vi "ProducerConsumerData 1.vi"() -> ()   [LabVIEW 2017, in "Status Monitor Library.lvlib"]
doc: "Use this template to build a producer/consumer design pattern. Use this template when you need to execute a process, such as data analysis, when a data source, such as a triggered acquisition, produces data at an uneven rate and you need to execute the process when the data becomes available."
uses:
  Status Monitor Library.lvlib
  Communications/Communications Library.lvlib
panel:
  in  "Process Stop Button":bool
  out "Demuxing":bool
  out "Total Samples":i32
  out "Post-Buffered Samples":i32
  out "Pre-Buffered Samples":i32
  out "Device State":T1(ring)
  in  "timeout (ms)":i32
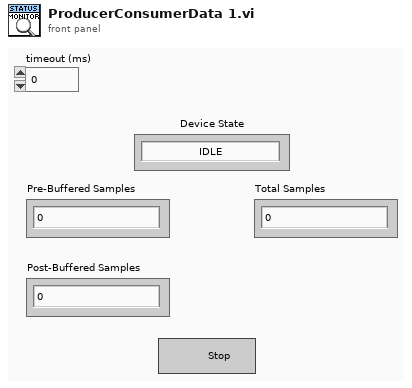
[diagram p1: front panel]
types:
  T1 = enum16{"IDLE", "ARM", "RUN_PRE-TRIGGER", "RUN_POST-TRIGGER", "POST_PROCESS", "CLEANUP"}
  T2 = typedef "Communications Library.lvlib/DTACQ Connection Data--Cluster.ctl" = cluster{"Description":string, "Address":string, "Port":u16, "timeout (ms)":i32, "Termination Character":string, "TCP Connection Reference":refnum<k5>, "Open Connection":bool}
  T3 = typedef "Communications Library.lvlib/DTACQ Module Carrier Status.ctl" = cluster{"DTACQ State":T4, "Pre-Trigger Samples":i32, "Post-Trigger Samples":i32, "Total Samples":i32, "Post Processing":bool}
  T4 = typedef "Communications Library.lvlib/DTACQ Status--Enum.ctl" = enum16{"IDLE", "ARM", "RUN_PRE-TRIGGER", "RUN_POST-TRIGGER", "POST_PROCESS", "CLEANUP"}
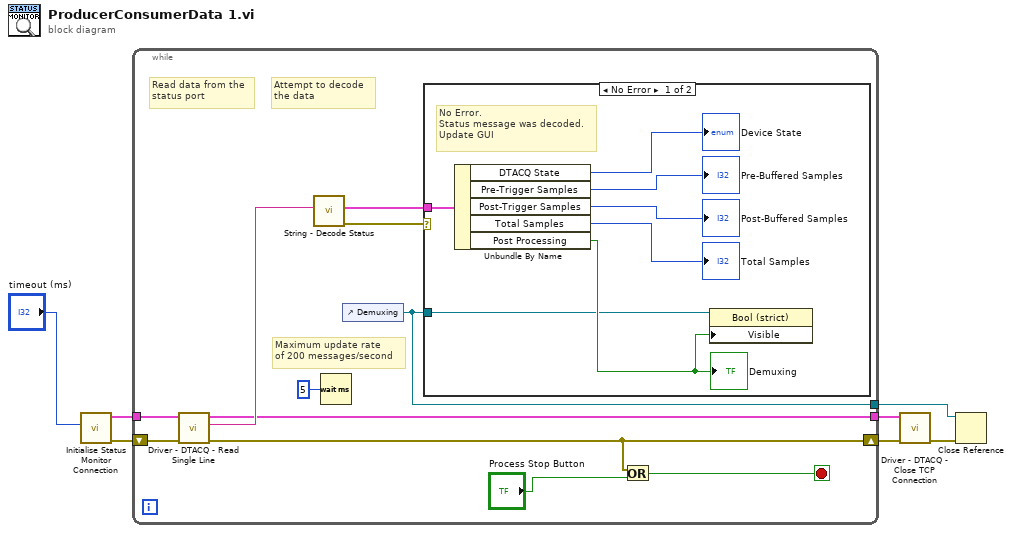
[diagram p0: block diagram]
diagram:
  n1 = call "Initialise Status Monitor Connection.vi"("timeout (ms)"="timeout (ms)") -> ("error out"=w5:errorcluster, "Status Connection Out"=w6:T2)  [unwired: 9 in]
  n2 = while {
    tunnel: w6 -> [w18]
    shift-right: [w13] -> w3
    shift-left: w5 -> [w16]
    tunnel: [w10] -> w4
    tunnel: [w9] -> w2
    stop <- w12 stop-if-true
    # "Maximum update rate\nof 200 messages/second"
    # "Attempt to decode\nthe data"
    # "Read data from the\nstatus port"
    n3 = call "Driver - DTACQ - Read Single Line.vi"("error in"=w16, "DTACQ Connection Data In"=w18) -> ("error out"=w13:errorcluster, "Read String"=w17:string, "DTACQ Connection Data Out"=w9:T2)  [unwired: 6 in, 1 out]
    n4 = call "String - Decode Status.vi"("Status Response String"=w17) -> ("error out"=w15:errorcluster, "Module Carrier Status"=w14:T3)  [unwired: 9 in]
    n5 = Wait (ms)(milliseconds to wait=u32 5) -> ()  [unwired: 1 out]
    n6 = control-ref of="Demuxing"() -> (w10:refnum<vi>)
    n7 = case shown="No Error" w15 {
      tunnel: w14 -> [w25 _]
      tunnel: w10 -> [w19 _]
      frame No Error {
        # "No Error.\nStatus message was decoded.\nUpdate GUI"
        n8 = Unbundle By Name(w25) -> ("DTACQ State"=→"Device State":T4, "Pre-Trigger Samples"=→"Pre-Buffered Samples":i32, "Post-Trigger Samples"=→"Post-Buffered Samples":i32, "Total Samples"=→"Total Samples":i32, "Post Processing"=w20:bool)
        "Demuxing" <- w20
        n9 = property class="Bool (strict)"(reference=w19, "Visible"=w20) -> ()  [unwired: 1 in, 2 out]
      }
      frame Error {
        # "Error decoding message.\nNot a valid status message,\nso leave the GUI as-is"
      }
    }
    n10 = Or(x=w13, y="Process Stop Button") -> (x .or. y?=w12:bool)
  }
  n11 = call "Driver - DTACQ - Close TCP Connection.vi"("error in"=w3, "DTACQ Connection Data In"=w2) -> ("error out"=w1:errorcluster)  [unwired: 8 in, 1 out]
  n12 = Close Reference(reference=w4, error in (no error)=w1) -> ()  [unwired: 1 out]
